vi "Func-패킷 프로토콜-패킷 분해.vi"(6 "ID":u32=2 format="%04x", 7 "메시지 데이터":string="\u00020202ss\u00031122") -> (1 "나머지 데이터":string="1122", 2 "메시지 데이터(Hex)":string="ss", 3 "패킷 정상":bool=TRUE)   [LabVIEW 2015]
panel:
  out "ID(in)":u32=2 format="%02x"
  out "패킷 데이터":string
  out "ETX":u32=3 format="%02x"
  out "STX":u32=2 format="%02x"
  out "패킷 전체 길이(바이트)":i32=12
  out "메시지 데이터 길이":u8=2 format="%.0x"
  # "* 패킷 프로토콜 - 프레임 데이터 전송"
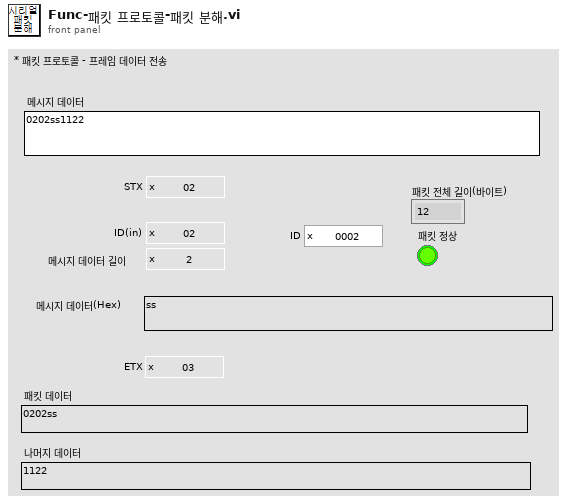
[diagram p1: front panel]
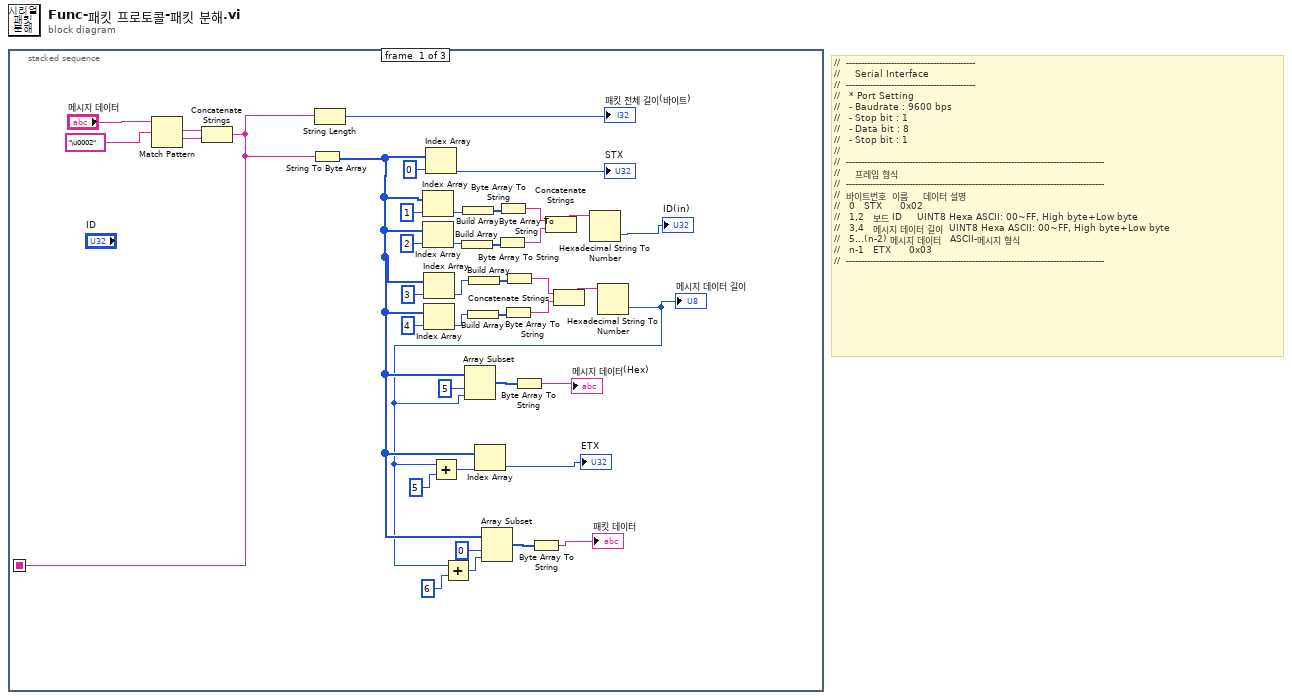
[diagram p0: block diagram]
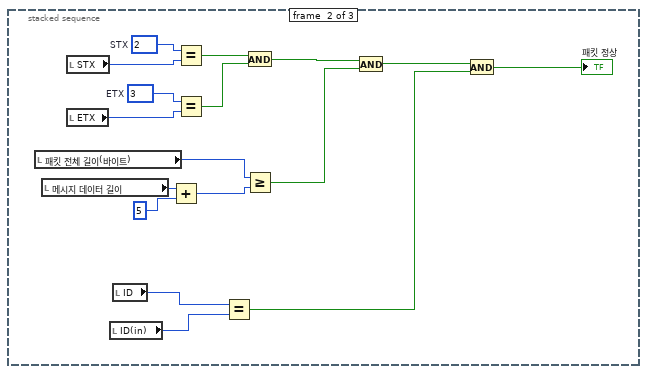
[diagram p2: hidden frame]
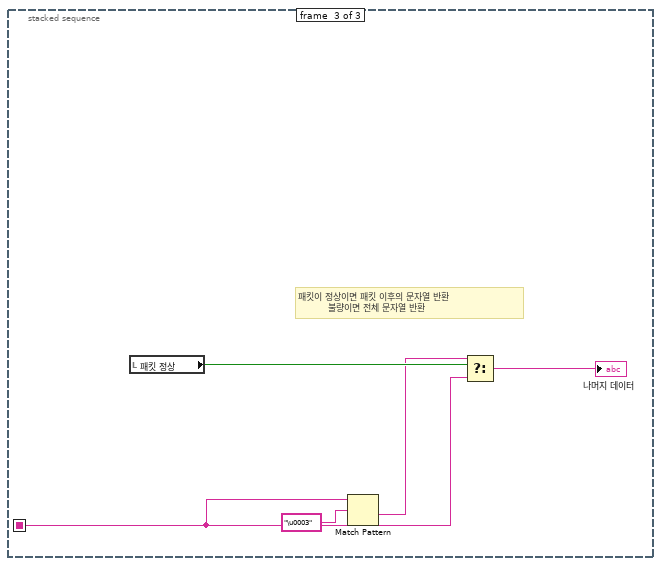
[diagram p3: hidden frame]
diagram:
  # "//\t\t-------------------------------------------\n//\t\t\t\t\tSerial Interface\n//\t\t-------------------------------------------\n//\t\t\t* Port Setting\n//\t\t\t- Baudrate : 9600 bps\n//\t\t\t- Stop bit : 1\n//\t\t\t- Data bit : 8 \n//\t\t\t- Stop bit : 1\t\n//\n//\t\t--------------------------------------------------------------------------------------\n//\t\t\t\t\t프레임 형식\n//\t\t--------------------------------------------------------------------------------------\n//\t\t바이트번호\t\t이름\t\t\t\t\t데이터 설명\n//\t\t\t0\t\t\tSTX \t\t\t\t\t0x02\n//\t\t\t1,2\t\t\t보드 ID \t\t\t\tUINT8 Hexa ASCII: 00~FF, High byte+Low byte\n//\t\t\t3,4\t\t\t메시지 데이터 길이\t\tUINT8 Hexa ASCII: 00~FF, High byte+Low byte\n//\t\t\t5...(n-2)\t메시지 데이터\t\t\tASCII-메시지 형식\n//\t\t\tn-1\t\t\tETX \t\t\t\t\t0x03\n//\t\t--------------------------------------------------------------------------------------"
  n1 = stacked-sequence {
    seq-local: [w28 _ _] -> [_ _ w59]
    frame #0 {
      n2 = Match Pattern(string="메시지 데이터", regular expression="\u0002") -> (match substring=w33:string, after substring=w32:string)  [unwired: 1 in, 2 out]
      n3 = Concatenate Strings(w33, w32) -> (w28:string)
      n4 = String To Byte Array(string=w28) -> (unsigned byte array=w20:u8[])
      n5 = String Length(string=w28) -> (length=→"패킷 전체 길이(바이트)":i32)
      n6 = Index Array(array=w20, index=1 ("인덱스")) -> (element=w16:u8)
      n7 = Index Array(array=w20, index=2 ("인덱스")) -> (element=w13:u8)
      n8 = Index Array(array=w20, index=3 ("인덱스")) -> (element=w10:u8)
      n9 = Index Array(array=w20, index=4 ("인덱스")) -> (element=w9:u8)
      n10 = Index Array(array=w20, index=0 ("인덱스")) -> (element=→"STX":u8)
      n11 = Build Array(w13) -> (w14:u8[])
      n12 = Build Array(w16) -> (w15:u8[])
      n13 = Build Array(w9) -> (w12:u8[])
      n14 = Build Array(w10) -> (w11:u8[])
      n15 = Byte Array To String(unsigned byte array=w14) -> (string=w6:string)
      n16 = Byte Array To String(unsigned byte array=w15) -> (string=w7:string)
      n17 = Byte Array To String(unsigned byte array=w12) -> (string=w2:string)
      n18 = Byte Array To String(unsigned byte array=w11) -> (string=w3:string)
      n19 = Concatenate Strings(w7, w6) -> (w8:string)
      n20 = Concatenate Strings(w3, w2) -> (w4:string)
      n21 = Hexadecimal String To Number(string=w8) -> (number=→"ID(in)":u32)  [unwired: 2 in, 1 out]
      n22 = Hexadecimal String To Number(string=w4) -> (number=w1:u32)  [unwired: 2 in, 1 out]
      "메시지 데이터 길이" <- w1
      n23 = Add(x=w1, y=5 ("인덱스")) -> (x+y=w23:u32)
      n24 = Add(x=w1, y=6 ("인덱스")) -> (x+y=w17:u32)
      n25 = Array Subset(array=w20, index=5 ("인덱스"), length=w1) -> (w30:u8[])
      n26 = Index Array(array=w20, index=w23) -> (element=→"ETX":u8)
      n27 = Array Subset(array=w20, index=0 ("인덱스"), length=w17) -> (w22:u8[])
      n28 = Byte Array To String(unsigned byte array=w30) -> (string=→"메시지 데이터(Hex)":string)
      n29 = Byte Array To String(unsigned byte array=w22) -> (string=→"패킷 데이터":string)
    }
    frame #1 {
      w54 = u8 3  # ETX
      w56 = u8 2  # STX
      n30 = local read "패킷 전체 길이(바이트)"() -> (w48:i32)
      n31 = local read "메시지 데이터 길이"() -> (w51:u8)
      n32 = local read "STX"() -> (w57:u32)
      n33 = local read "ETX"() -> (w55:u32)
      n34 = local read "ID(in)"() -> (w44:u32)
      n35 = local read "ID"() -> (w45:u32)
      n36 = Add(x=w51, y=u32 5) -> (x+y=w49:u32)
      n37 = Equal?(x=w56, y=w57) -> (x = y?=w53:bool)
      n38 = Equal?(x=w54, y=w55) -> (x = y?=w52:bool)
      n39 = Equal?(x=w45, y=w44) -> (x = y?=w42:bool)
      n40 = And(x=w53, y=w52) -> (x .and. y?=w47:bool)
      n41 = Greater Or Equal?(x=w48, y=w49) -> (x >= y?=w46:bool)
      n42 = And(x=w47, y=w46) -> (x .and. y?=w43:bool)
      n43 = And(x=w43, y=w42) -> (x .and. y?=→"패킷 정상":bool)
    }
    frame #2 {
      # "패킷이 정상이면 패킷 이후의 문자열 반환\n          불량이면 전체 문자열 반환"
      n44 = local read "패킷 정상"() -> (w62:bool)
      n45 = Match Pattern(string=w59, regular expression="\u0003") -> (after substring=w58:string)  [unwired: 1 in, 3 out]
      n46 = Select(t=w58, s=w62, f=w59) -> (s? t:f=→"나머지 데이터":string)
    }
  }
